vi "PID Turn.vi"(9 "Reset gyro":bool, 10 "Error Tolerance +/- (3)":dbl=2.5, 11 "Setpoint":dbl) -> (3 "Angel out":dbl)   [LabVIEW 2015]
uses:
  <vilib>/addons/control/pid/pid.llb/PID Structure Conversion (DBL).vi
  <vilib>/Rock Robotics/WPI/Utilities/WPI_GetSetVariantRefNum.vi
  <vilib>/addons/control/pid/pid.llb/PID Control Input Filter (DBL).vi
  <vilib>/addons/control/pid/pid.llb/PID (DBL).vi
  <vilib>/addons/control/pid/NI_PID_pid.lvlib
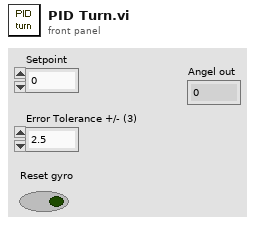
[diagram p1: front panel]
types:
  T1 = cluster{"proportional gain (Kc)":dbl, "integral time (Ti, min)":dbl, "derivative time (Td, min)":dbl}
  T2 = typedef "WPI_GyroDevRef.ctl" = cluster{"DevStatus":errorcluster, "Analog Channel":T3, "Offset":dbl, "Gain (VoltsPerDegree/Second)":dbl, "Gyro Type":enum16{"Analog", "XRS450"}, "Handle":i32, "SPI Bus":T4, "Device Found":bool, "Sample Rate":dbl, "Calibrate On Open":bool}
  T3 = typedef "FPGA_AIChannel.ctl" = enum8{"AI 0", "AI 1", "AI 2", "AI 3", "AI MXP 0", "AI MXP 1", "AI MXP 2", "AI MXP 3", "Invalid"}
  T4 = typedef "spi_bus.ctl" = enum16{"SPI On-Board, CS0", "SPI On-Board, CS1", "SPI On-Board, CS2", "SPI On-Board, CS3", "SPI MXP", "Invalid"}
  T5 = typedef "WPI_RobotDriveDevRef.ctl" = cluster{"DevStatus":errorcluster, "Motors[]":T6[], "Square Inputs":bool, "Max Output":dbl}
  T6 = typedef "WPI_MotorControlDeviceRef.ctl" = cluster{"DeviceStatus":errorcluster, "Type":T7, "PWM":cluster{"PWM Channel":T8, "DeadBand":T9}, "CAN":cluster{"Device Number":u8, "Control Mode":T10, "Semaphore":T11, "Max Vout":dbl, "TalonSRX Control Mode":T12}, "Invert":bool}
  T7 = typedef "WPI_MotorControlType.ctl" = enum16{"PWM", "CAN", "CANTalonSRX"}
  T8 = typedef "FPGA_DIOPWMChannel.ctl" = enum8{"PWM 0", "PWM 1", "PWM 2", "PWM 3", "PWM 4", "PWM 5", "PWM 6", "PWM 7", "PWM 8", "PWM 9", "PWM MXP 0", "PWM MXP 1", "PWM MXP 2", "PWM MXP 3", "PWM MXP 4", "PWM MXP 5", "PWM MXP 6", "PWM MXP 7", "PWM MXP 8", "PWM MXP 9", "Invalid"}
  T9 = typedef "WPI_PWMDeadband.ctl" = cluster{"Name":string, "maxPositivePwm":i32, "minPositivePwm":i32, "centerPwm":i32, "maxNegativePwm":i32, "minNegativePwm":i32, "angularRange":u16}
  T10 = typedef "WPI_CANJaguar_ControlMode.ctl" = enum8{"Percent VBus", "Current", "Speed", "Position", "Voltage"}
  T11 = typedef "Semaphore RefNum" = refnum<k1>
  T12 = typedef "WPI_CANTalonSRX_APIControlMode.ctl" = enum8{"Percent VBus", "Speed", "Position", "Slave", "Unchanged / Invalid", "Voltage Compensation", "Current", "Motion Profile"}
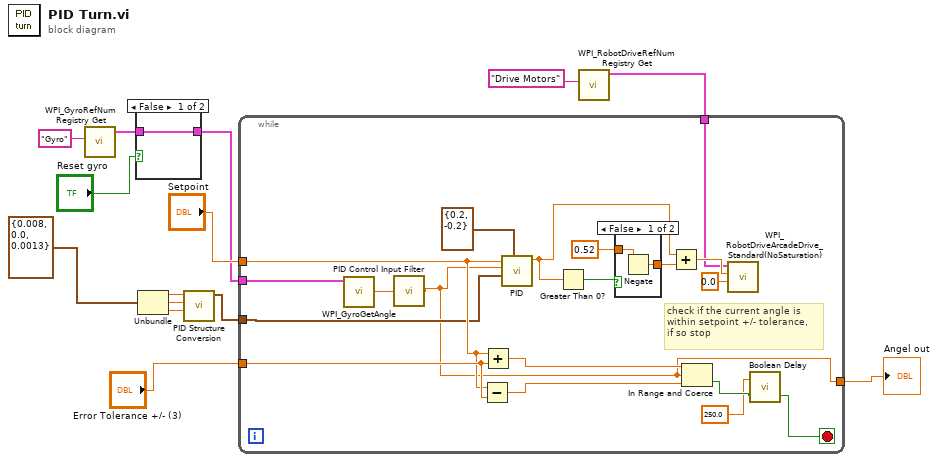
[diagram p0: block diagram]
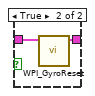
[diagram p2: hidden frame]
diagram:
  n1 = call <vilib>:"WPI_GyroRefNum Registry Get.vi"("refnum name"="Gyro") -> ("GyroDevRef"=w4:T2)  [unwired: 9 in, 1 out]
  n2 = case shown="False" "Reset gyro" {
    tunnel: w4 -> [w15 w17]
    tunnel: [w15 w16] -> w3
    frame False {
    }
    frame True {
      n3 = call <vilib>:"WPI_GyroReset.vi"("GyroDevRef"=w17) -> ("GyroDevRef"=w16:T2)  [unwired: 9 in, 1 out]
    }
  }
  n4 = Unbundle(T1 {"proportional gain (Kc)"=0.008, "integral time (Ti, min)"=0.0, "derivative time (Td, min)"=0.0013} ("PID gains")) -> ("proportional gain (Kc)"=w12:dbl, "integral time (Ti, min)"=w13:dbl, "derivative time (Td, min)"=w14:dbl)
  n5 = call-poly <vilib>:"PID Structure Conversion.vi"("derivative"=w14, "integral"=w13, "proportional"=w12) -> ("PID gains"=w9:T1)  [unwired: 8 in]
  n6 = call <vilib>:"WPI_RobotDriveRefNum Registry Get.vi"("refnum name"="Drive Motors") -> ("RobotDriveDevRef"=w6:T5)  [unwired: 1 in, 9 out]
  n7 = while {
    tunnel: "Setpoint" -> [w31]
    tunnel: w9 -> [w30]
    tunnel: "Error Tolerance +/- (3)" -> [w32]
    tunnel: w6 -> [w23]
    tunnel: w3 -> [w22]
    tunnel: [w21] -> w1
    stop <- w19 stop-if-true
    # "check if the current angle is\nwithin setpoint +/- tolerance,\nif so stop"
    n8 = call <vilib>:"WPI_GyroGetAngle.vi"("GyroDevRef"=w22) -> ("Angle"=w24:dbl)  [unwired: 6 in, 4 out]
    n9 = call-poly <vilib>:"PID Control Input Filter.vi"("input"=w24) -> ("output"=w21:dbl)  [unwired: 4 in]
    n10 = Subtract(x=w31, y=w32) -> (x-y=w33:dbl)
    n11 = Add(x=w31, y=w32) -> (x+y=w34:dbl)
    n12 = call-poly <vilib>:"PID.vi"("output range"=cluster{"output high":dbl, "output low":dbl} {"output high"=0.2, "output low"=-0.2}, "PID gains"=w30, "process variable"=w21, "setpoint"=w31) -> ("output"=w28:dbl)  [unwired: 6 in, 1 out]
    n13 = Greater Than 0?(x=w28) -> (x > 0?=w29:bool)
    n14 = case shown="False" w29 {
      tunnel: [w37 w39] -> w27
      tunnel: 0.52 -> [w38 w39]
      frame False {
        n15 = Negate(x=w38) -> (-x=w37:dbl)
      }
      frame True {
      }
    }
    n16 = Add(x=w28, y=w27) -> (x+y=w25:dbl)
    n17 = In Range and Coerce(upper limit=w34, x=w21, lower limit=w33) -> (In Range?=w20:bool)  [unwired: 1 out]
    n18 = call <vilib>:"WPI_RobotDriveArcadeDrive_Standard(NoSaturation).vi"("Y axis value"=0.0, "X axis value"=w25, "RobotDriveDevRef"=w23) -> ()  [unwired: 1 in, 8 out]
    n19 = call "Boolean Delay.vi"("Input"=w20, "Delay (ms)"=250.0) -> ("Output"=w19:bool)  [unwired: 1 in]
  }
  "Angel out" <- w1
